vi "Contador_de_pulsos_horario_y_Antihorario.vi"() -> ()   [LabVIEW 2025]
panel:
  in  "Posición cero":bool
  out "Pulsos":dbl
  out "Sentido de giro":string
  in  "stop":bool
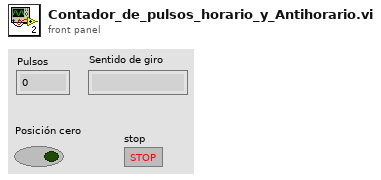
[diagram p1: front panel]
types:
  T1 = enum16{"Estado Defecto", "Estado 1", "Estado 2", "Estado 3"}
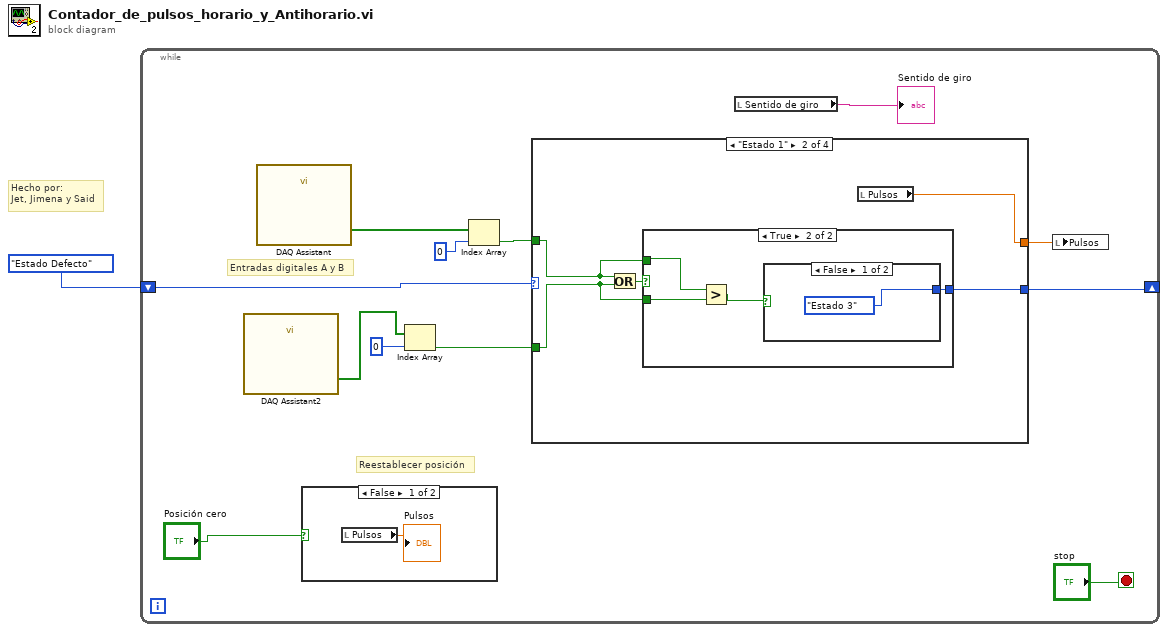
[diagram p0: block diagram]
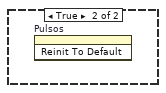
[diagram p2: hidden frame]
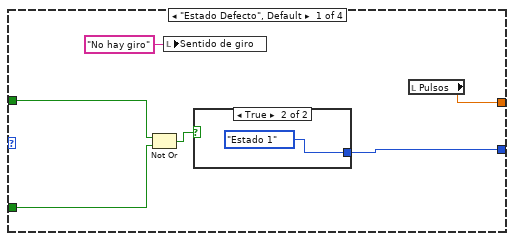
[diagram p3: hidden frame]
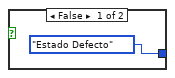
[diagram p4: hidden frame]
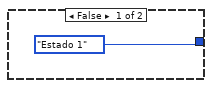
[diagram p5: hidden frame]
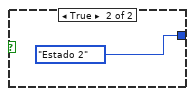
[diagram p6: hidden frame]
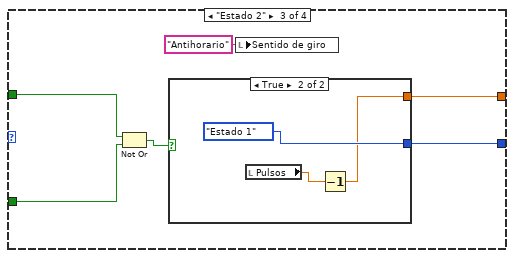
[diagram p7: hidden frame]
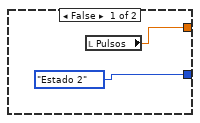
[diagram p8: hidden frame]
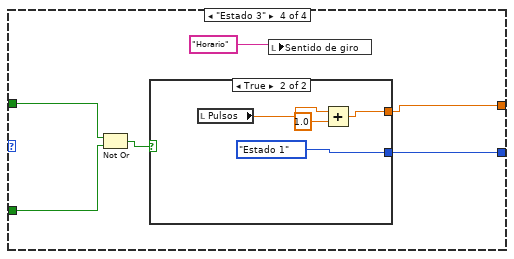
[diagram p9: hidden frame]
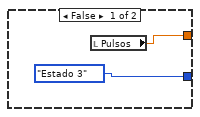
[diagram p10: hidden frame]
diagram:
  # "Hecho por:\nJet, Jimena y Said"
  n1 = while {
    shift-right: [w12] -> _
    shift-left: T1."Estado Defecto" -> [w13]
    stop <- "stop" stop-if-true
    # "Reestablecer posición"
    # "Entradas digitales A y B"
    n2 = call "DAQ Assistant2"() -> ("data"=w3:bool[])  [unwired: 17 in, 2 out]
    n3 = call "DAQ Assistant"() -> ("data"=w2:bool[])  [unwired: 17 in, 2 out]
    n4 = case shown="False" "Posición cero" {
      frame False {
        n5 = local read "Pulsos"() -> (→"Pulsos":dbl)
      }
      frame True {
        n6 = invoke on="Pulsos" class="DigNum (strict)" method="Reinit To Default"() -> ()  [unwired: 3 in, 3 out]
      }
    }
    n7 = Index Array(array=w3, index=0) -> (element=w9:bool)
    n8 = Index Array(array=w2, index=0) -> (element=w6:bool)
    n9 = case shown="\"Estado 1\"" w13 {
      tunnel: [w19 w26 w39 w50] -> w12
      tunnel: w9 -> [w15 w23 w35 w46]
      tunnel: w6 -> [w16 w24 w36 w47]
      tunnel: [w17 w25 w37 w48] -> w8
      frame "Estado Defecto", Default {
        n10 = Not Or(1:w15, 2:w16) -> (0:w20:bool)
        n11 = local write "Sentido de giro"("No hay giro" ("Sentido de giro")) -> ()
        n12 = case shown="True" w20 {
          tunnel: [T1."Estado Defecto" T1."Estado 1"] -> w19
          frame False {
          }
          frame True {
          }
        }
        n13 = local read "Pulsos"() -> (w17:dbl)
      }
      frame "Estado 1" {
        n14 = Or(x=w24, y=w23) -> (x .or. y?=w27:bool)
        n15 = case shown="True" w27 {
          tunnel: [T1."Estado 1" w31] -> w26
          tunnel: w24 -> [_ w30]
          tunnel: w23 -> [_ w29]
          frame False {
          }
          frame True {
            n16 = Greater?(x=w30, y=w29) -> (0:w32:bool)
            n17 = case shown="False" w32 {
              tunnel: [T1."Estado 3" T1."Estado 2"] -> w31
              frame False {
              }
              frame True {
              }
            }
          }
        }
        n18 = local read "Pulsos"() -> (w25:dbl)
      }
      frame "Estado 2" {
        n19 = Not Or(1:w35, 2:w36) -> (0:w40:bool)
        n20 = case shown="True" w40 {
          tunnel: [T1."Estado 2" T1."Estado 1"] -> w39
          tunnel: [w41 w43] -> w37
          frame False {
            n21 = local read "Pulsos"() -> (w41:dbl)
          }
          frame True {
            n22 = local read "Pulsos"() -> (w44:dbl)
            n23 = Decrement(x=w44) -> (x-1=w43:dbl)
          }
        }
        n24 = local write "Sentido de giro"("Antihorario") -> ()
      }
      frame "Estado 3" {
        n25 = Not Or(1:w46, 2:w47) -> (0:w51:bool)
        n26 = case shown="True" w51 {
          tunnel: [T1."Estado 3" T1."Estado 1"] -> w50
          tunnel: [w52 w55] -> w48
          frame False {
            n27 = local read "Pulsos"() -> (w52:dbl)
          }
          frame True {
            n28 = local read "Pulsos"() -> (w54:dbl)
            n29 = Add(x=w54, y=1.0) -> (x+y=w55:dbl)
          }
        }
        n30 = local write "Sentido de giro"("Horario") -> ()
      }
    }
    n31 = local read "Sentido de giro"() -> (→"Sentido de giro":string)
    n32 = local write "Pulsos"(w8) -> ()
  }
